vi "Fpga-Feedback-Test.vi"   [LabVIEW 2017]
uses:
  <vilib>/Platform/TimedLoop/XDataNode/timing_clust.ctl
  <vilib>/Platform/TimedLoop/XDataNode/nitl_modes.ctl
  <vilib>/Platform/TimedLoop/XDataNode/wakeup.ctl
  <vilib>/rvi/Emulation/niFpgaSctlEmulationGetInTimedLoop.vi
  <vilib>/rvi/Emulation/niFpgaEmulationReportErrorSimple.vi
  <vilib>/rvi/Emulation/niFpgaGetClockAttributes.vi
  <vilib>/rvi/Emulation/niFpgaCriticalErrorInLSC.vi
  <vilib>/rvi/interface/RandomDataEmulation/niFpgaRandomDataHandleErrors.vi
  <vilib>/Platform/TimedLoop/XDataNode/XDataNode.xnode
  <vilib>/rvi/DataTransferAndStorage/Container/XNode/niFpgaContainer.xnode
  <vilib>/rvi/interface/RandomDataEmulation/nirviRandomDataFpgaReadWriteTemplate.vi
  <vilib>/Platform/TimedLoop/XDataNode/XDNodeRunTimeDep.lvlib
types:
  T1 = typedef "XDNodeRunTimeDep.lvlib/timing_clust.ctl" = cluster{"Expected End [f-1]":u64, "Actual End [f-1]":u64, "Finished Late? [f-1]":bool, "Expected End [i-1]":u64, "Actual End [i-1]":u64, "Finished Late? [i-1]":bool, "Expected Start [i]":u64, "Actual Start [i]":u64, "Expected Start [f]":u64, "Actual Start [f]":u64, "Source Name":string, "Structure Name":string, "Period":i64, "Deadline":i64, "Offset":i64, "Start":i64, "Priority":i32, "Timeout":i32, "Mode":T2, "Wakeup Reason":T3, "Error":errorcluster, "Source Type":string, "Secondary Source Type":string, "Global End Time":u64, "Global Start Time":u64, "Frame Duration":u64, "Iteration Duration":u64, "Assigned CPU":i32, "I/O Scan Engine Mode":u32}
  T2 = typedef "XDNodeRunTimeDep.lvlib/nitl_modes.ctl" = enum32{"No Change", "Process missed periods, maintain original phase", "Discard missed periods, maintain original phase", "Process missed periods, ignore original phase", "Discard missed periods, ignore original phase"}
  T3 = typedef "XDNodeRunTimeDep.lvlib/wakeup.ctl" = enum32{"Normal", "Aborted", "Asynchronous wakeup", "Timing source error", "Timed loop error", "Timeout"}
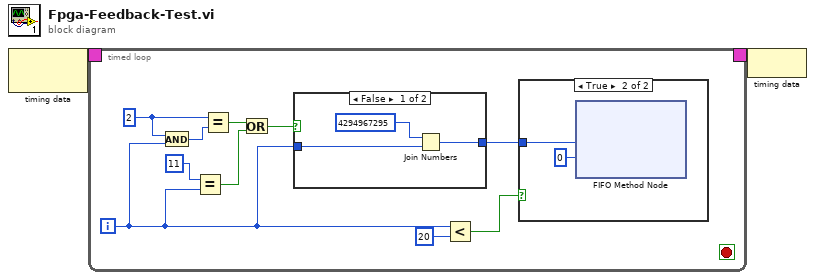
[diagram p0: block diagram]
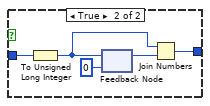
[diagram p3: hidden frame]
diagram:
  n1 = node-c288() -> (w2:T1)  [unwired: 1 in]
  n2 = timed-loop {
    timing: w2 -> [_]
    timing-out: [_] -> w1
    i -> [w6]
    stop <- _ stop-if-true
    w11 = 2 ("x")
    n3 = And(x=w11, y=w6) -> (x .and. y?=w12:i32)
    n4 = Equal?(x=11, y=w6) -> (x = y?=w8:bool)
    n5 = Equal?(x=w11, y=w12) -> (x = y?=w10:bool)
    n6 = Or(x=w10, y=w8) -> (x .or. y?=w7:bool)
    n7 = case shown="False" w7 {
      tunnel: w6 -> [w15 w19]
      tunnel: [w17 w20] -> w4
      frame False {
        n8 = Join Numbers(hi=u32 4294967295, lo=w15) -> ((hi.lo)=w17:u64)
      }
      frame True {
        n9 = To Unsigned Long Integer(number=w19) -> (unsigned 32bit integer=w18:u32)
        n10 = feedback-in #1(w18) -> ()
        n11 = feedback #1(u32 0) -> (w21:u32)
        n12 = Join Numbers(hi=w18, lo=w21) -> ((hi.lo)=w20:u64)
      }
    }
    n13 = Less?(x=w6, y=20) -> (x < y?=w3:bool)
    n14 = case shown="True" w3 {
      tunnel: w4 -> [_ w14]
      frame False {
      }
      frame True {
        n15 = xnode ("FIFO Method Node")("Element"=w14, "Timeout"=0) -> ()  [unwired: 1 in, 2 out]
      }
    }
  }
  n16 = node-c288(w1) -> ()
